vi "Read Faults.vi"(8 "error in (no error)":errorcluster, 11 "MKS MW in":refnum<class "PL MKS MW.lvclass">) -> (0 "error out":errorcluster, 2 "faults":T1, 3 "MKS MW out":refnum<class "PL MKS MW.lvclass">)   [LabVIEW 2015, in "PL MKS MW.lvclass"]
doc: "Reads device status (faults)."
uses:
  PL MKS MW.lvclass
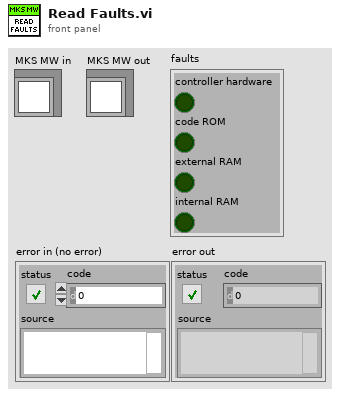
[diagram p1: front panel]
types:
  T1 = cluster{"controller hardware":bool, "code ROM":bool, "external RAM":bool, "internal RAM":bool}
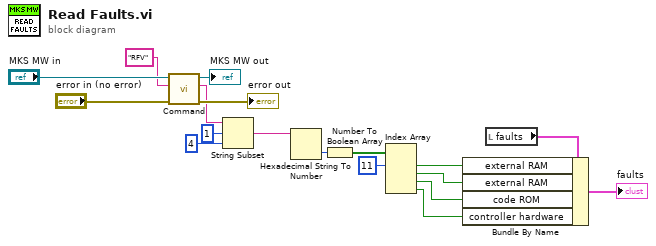
[diagram p0: block diagram]
diagram:
  n1 = call "Command.vi"("error in (no error)"="error in (no error)", "command"="RFV", "MKS MW in"="MKS MW in") -> ("error out"=→"error out":errorcluster, "response data"=w11:string, "MKS MW out"=→"MKS MW out":refnum<class "PL MKS MW.lvclass">)  [unwired: 6 in]
  n2 = String Subset(string=w11, offset (0)=1, length (rest)=4 ("length (rest)")) -> (substring=w4:string)
  n3 = Hexadecimal String To Number(string=w4) -> (number=w10:u32)  [unwired: 2 in, 1 out]
  n4 = Number To Boolean Array(number=w10) -> (Boolean array=w1:bool[])
  n5 = Index Array(array=w1, index #1=11 ("index")) -> (element #1=w8:bool, element #2=w7:bool, element #3=w6:bool, element #4=w5:bool)  [unwired: 3 in]
  n6 = local read "faults"() -> (w13:T1)
  n7 = Bundle By Name(cluster=w13, "external RAM"=w8, "external RAM"=w7, "code ROM"=w6, "controller hardware"=w5) -> (→"faults":T1)
